vi "GetFPNamesAndLocns.vi"() -> (2 "Array":T1[](array[typedef]))   [LabVIEW 2020]
uses:
  Anemometry Sub Vis/Controls/VInameSizePath.ctl
  <vilib>/Utility/miscctls.llb/LVRectTypeDef.ctl
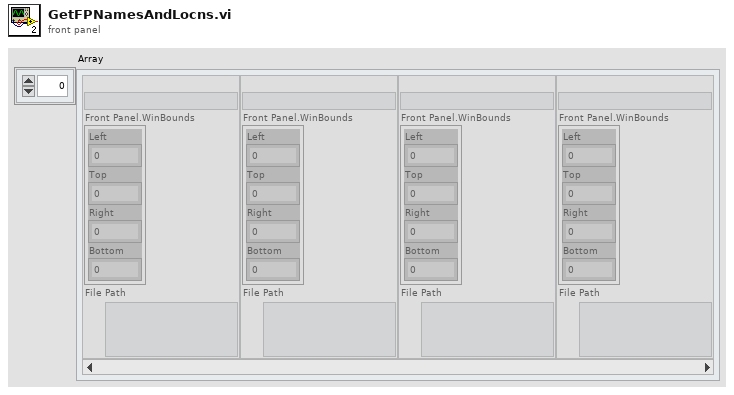
[diagram p1: front panel]
types:
  T1 = typedef "VInameSizePath.ctl" = cluster{"VI Name":string, "Front Panel.WinBounds":T2, "File Path":path}
  T2 = typedef "LVRectTypeDef.ctl" = cluster{"Left":i16, "Top":i16, "Right":i16, "Bottom":i16}
  T3 = typedef "VIMemory VI info.ctl" = cluster{"Project":string, "ComputingNode":string, "VI Name":string, "App Refnum":refnum<vi>}
  T4 = cluster{"VI Name":string, "Front Panel.WinBounds":T2, "Path":path}
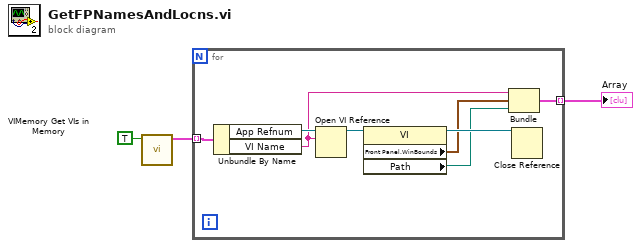
[diagram p0: block diagram]
diagram:
  n1 = call <vilib>:"VIMemory Get VIs in Memory.vi"("Only VIs with Open FPs?"=TRUE) -> ("VIs in memory"=w2:T3[])  [unwired: 9 in, 1 out]
  n2 = for {
    tunnel: w2 -> [w9] mode=indexing
    tunnel: [w7] -> w1 mode=indexing
    n3 = Unbundle By Name(w9) -> ("App Refnum"=w8:refnum<vi>, "VI Name"=w6:string)
    n4 = Open VI Reference(application reference (local)=w8, vi path=w6) -> (vi reference=w11:refnum<vi>)  [unwired: 4 in, 1 out]
    n5 = property class="VI"(reference=w11) -> (reference out=w10:refnum<vi>, "Front Panel.WinBounds"=w5:T2, "Path"=w4:path)  [unwired: 1 in, 1 out]
    n6 = Bundle("VI Name"=w6, "Front Panel.WinBounds"=w5, "Path"=w4) -> (w7:T4)  [unwired: 1 in]
    n7 = Close Reference(reference=w10) -> ()  [unwired: 1 in, 1 out]
  }
  "Array" <- w1
